vi "closeViewer.vi"(8 "error in (no error)":errorcluster, 11 "ImageStreamViewer in":refnum<class "ImageStreamViewer.lvclass">) -> (0 "error out":errorcluster, 3 "ImageStreamViewer out":refnum<class "ImageStreamViewer.lvclass">)   [LabVIEW 2009, in "Views.lvlib" / "Camera.lvlib" / "ImageStreamViewer.lvclass"]
uses:
  ImageStreamViewer.lvclass
  ImageStreamViewer.lvclass/ImageStreamViewer.ctl
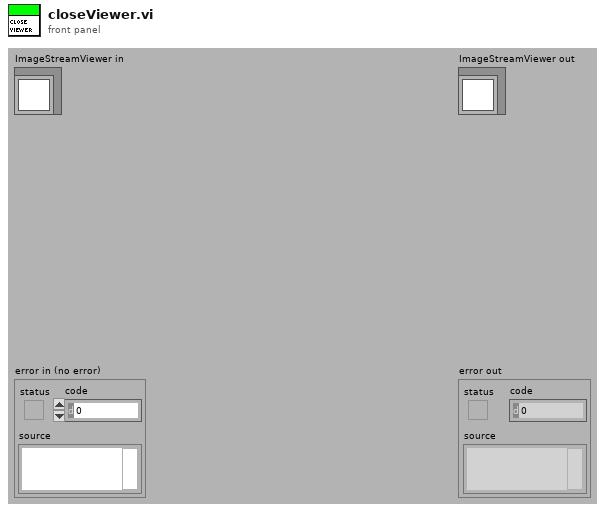
[diagram p1: front panel]
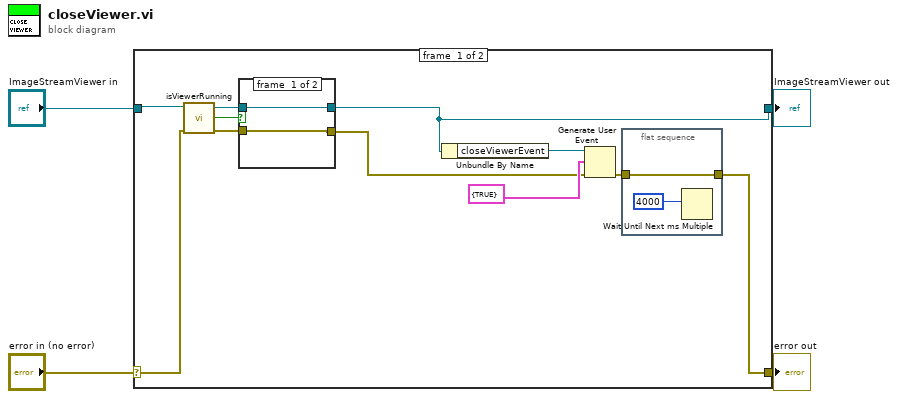
[diagram p0: block diagram]
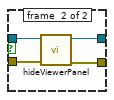
[diagram p2: hidden frame]
diagram:
  n1 = case shown="No Error" "error in (no error)" {
    selector: "error in (no error)" -> [w12 w25]
    tunnel: [w5 w25] -> w3
    tunnel: [w9 w24] -> w1
    tunnel: "ImageStreamViewer in" -> [w13 w24]
    frame #0 {
      n2 = call "isViewerRunning.vi"("error in (no error)"=w12, "ImageStreamViewer in"=w13) -> ("error out"=w11:errorcluster, "running?"=w7:bool, "ImageStreamViewer out"=w10:refnum<class "ImageStreamViewer.lvclass">)  [unwired: 7 in]
      n3 = case shown="True" w7 {
        tunnel: w11 -> [w18 w23]
        tunnel: w10 -> [w19 w22]
        tunnel: [w19 w21] -> w9
        tunnel: [w18 w20] -> w8
        frame #0 {
        }
        frame #1 {
          n4 = call "hideViewerPanel.vi"("error in (no error)"=w23, "ImageStreamViewer in"=w22) -> ("error out"=w20:errorcluster, "ImageStreamViewer out"=w21:refnum<class "ImageStreamViewer.lvclass">)  [unwired: 8 in]
        }
      }
      n5 = Unbundle By Name(w9) -> ("closeViewerEvent"=w15:refnum<user-event>)
      n6 = Generate User Event(user event=w15, event data cluster=cluster{bool} {TRUE} ("event data"), error in=w8) -> (error out=w6:errorcluster)  [unwired: 1 out]
      n7 = flat-sequence {
        tunnel: [w17] -> w5
        tunnel: w6 -> [w17]
        frame #0 {
          n8 = Wait Until Next ms Multiple(millisecond multiple=4000) -> ()  [unwired: 1 out]
        }
      }
    }
    frame #1 {
    }
  }
  "error out" <- w3
  "ImageStreamViewer out" <- w1
